vi "Clear Waypoint Route.vi"(8 "Error In":errorcluster, 9 "Main Map Reference":refnum<k24>, 10 "Main Map DLL Ref":refnum<k24>, 11 "Route Index":i32) -> (0 "error out":errorcluster)   [LabVIEW 2014]
uses:
  C:/Robotic Systems/Products/Surveyor/Software/Ground Station/Data/Mapping DLL/GMap.NET.WindowsForms.dll
  Data/Mapping DLL/GMap.NET.WindowsForms.dll
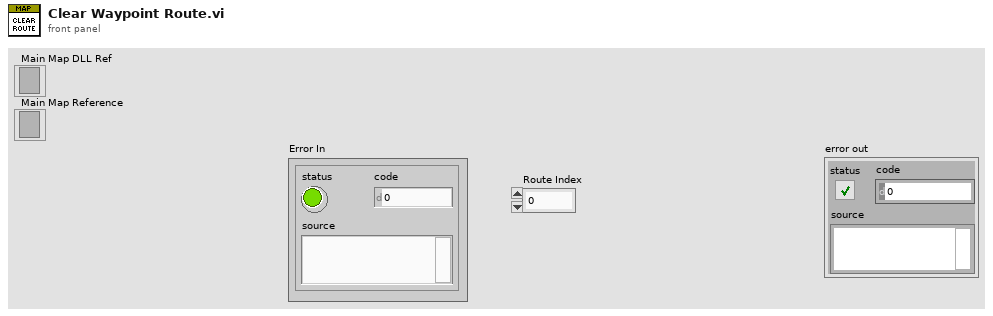
[diagram p1: front panel]
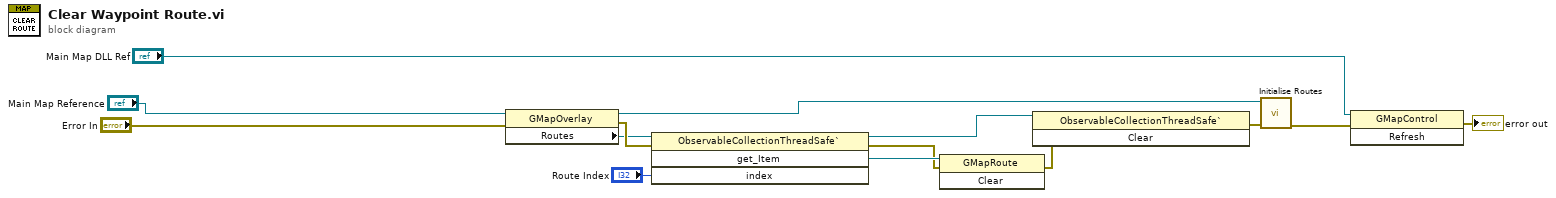
[diagram p0: block diagram]
diagram:
  n1 = property class="GMapOverlay"(reference="Main Map Reference", error in="Error In") -> (reference out=w4:refnum<k24>, error out=w14:errorcluster, "Routes"=w12:refnum<k24>)
  n2 = invoke class="ObservableCollectionThreadSafe`" method="get_Item"(reference=w12, error in=w14, "index"="Route Index") -> (reference out=w5:refnum<k24>, error out=w10:errorcluster, "get_Item"=w11:refnum<k24>)  [unwired: 1 in, 1 out]
  n3 = invoke class="GMapRoute" method="Clear"(reference=w11, error in=w10) -> (error out=w7:errorcluster)  [unwired: 1 in, 2 out]
  n4 = invoke class="ObservableCollectionThreadSafe`" method="Clear"(reference=w5, error in=w7) -> (error out=w6:errorcluster)  [unwired: 1 in, 2 out]
  n5 = call "Initialise Routes.vi"("error in (no error)"=w6, "Main Overlay"=w4) -> ("error out"=w8:errorcluster)  [unwired: 9 in]
  n6 = invoke class="GMapControl" method="Refresh"(reference="Main Map DLL Ref", error in=w8) -> (error out=→"error out":errorcluster)  [unwired: 1 in, 2 out]
